vi "周期任务设置.vi"(11 "TimingControl 输入":refnum<class "TimingControl.lvclass">) -> (3 "TimingControl 输出":refnum<class "TimingControl.lvclass">)   [LabVIEW 2016, in "TimingControl.lvlib" / "TimingControl.lvclass"]
uses:
  TimingControl.lvclass
  <vilib>/Utility/miscctls.llb/LVPointTypeDef.ctl
  TimingControl.lvclass/TimingControl.ctl
panel:
  in  "保存":bool
  in  "退出":bool
  in  "添加":bool
  in  "删除":bool
  in  "清空":bool
  in  "任务列表":i32(listbox)
  out "启动次数":i32
  out "测试状态.启动时间":timestamp caption="启动时间" format="%<%y/%m/%d %H:%M:%S>T"
  in  "每日启动":T1
  in  "每周启动":T2
  in  "每月启动":T3
  in  "控制命令":T4
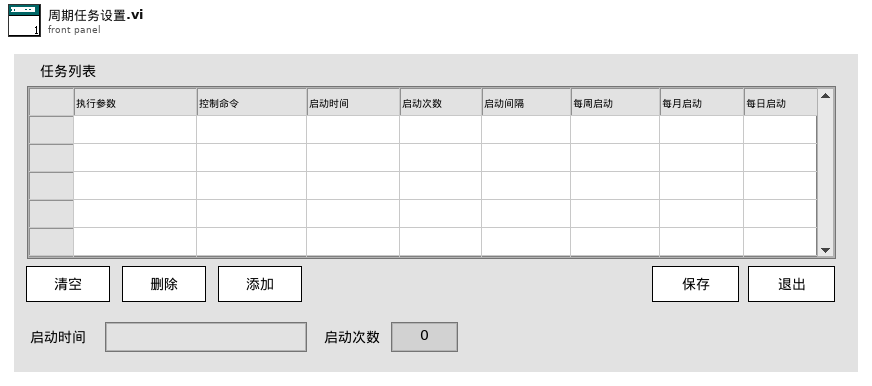
[diagram p1: front panel]
types:
  T1 = typedef "TimingControl.lvlib/TimingControl.lvclass/每日启动.ctl" = enum16{"关闭", "每日"}
  T2 = typedef "TimingControl.lvlib/TimingControl.lvclass/每周启动.ctl" = enum16{"关闭", "周日", "周一", "周二", "周三", "周四", "周五", "周六"}
  T3 = typedef "TimingControl.lvlib/TimingControl.lvclass/每月启动.ctl" = enum16{"关闭", "1号", "2号", "3号", "4号", "5号", "6号", "7号", "8号", "9号", "10号", "11号", "12号", "13号", "14号", "15号", "16号", "17号", "18号", "19号", "20号", "21号", "22号", "23号", "24号", "25号", "26号", "27号", "28号", "29号", "30号", "31号"}
  T4 = typedef "TimingControl.lvlib/TimingControl.lvclass/国标控制命令.ctl" = enum16{"启动测量", "标样核查", "零点核查", "跨度核查", "空白测试", "平行样测试", "加标回收", "空白校准", "标样校准", "初始化（清洗）", "停止测试", "仪器重启", "校时", "模式设置", "测量间隔设置"}
  T5 = typedef "LVPointTypeDef.ctl" = cluster{"Horizontal":i16, "Vertical":i16}
  T6 = typedef "TimingControl.lvlib/TimingControl.lvclass/State Data.ctl" = cluster{"仪器时间":timestamp, "仪器运行状态":bool, "配置文件路径":path, "测量参数":T7, "测试状态":cluster{"启动时间":timestamp, "结束时间":timestamp, "启动次数":i32}, "配置信息":T8}
  T7 = typedef "TimingControl.lvlib/TimingControl.lvclass/测量参数.ctl" = cluster{"测量参数":string[]}
  T8 = typedef "TimingControl.lvlib/TimingControl.lvclass/配置信息.ctl" = cluster{"每周启动":T2, "每月启动":T3, "周期模式":T9, "测量参数":T7, "定点周期":T10, "间隔启动":T12, "配置时间":timestamp, "配置":cluster{"测量参数":string, "控制命令":T4, "启动时间":string, "启动次数":u16, "启动间隔":dbl, "每周启动":T2, "每月启动":T3, "每日启动":enum16{"关闭", "每日"}}[]}
  T9 = typedef "TimingControl.lvlib/TimingControl.lvclass/周期模式设置.ctl" = enum16{"定点模式", "间隔模式"}
  T10 = typedef "TimingControl.lvlib/TimingControl.lvclass/定点周期设置.ctl" = cluster{"时间":u16, "启动命令":T11}
  T11 = typedef "TimingControl.lvlib/TimingControl.lvclass/启动命令选择.ctl" = enum16{"", "水样测试", "标样核查", "零点核查", "跨度核查", "空白测试", "平行样测试", "加标回收", "空白校准", "标样校准", "初始化(清洗)"}
  T12 = typedef "TimingControl.lvlib/TimingControl.lvclass/间隔启动设置.ctl" = cluster{"启动命令":T11, "启动间隔":dbl, "启动次数":i32}
  T13 = cluster{"测量参数":string, "控制命令":T4, "启动时间":string, "启动次数":u16, "启动间隔":dbl, "每周启动":T2, "每月启动":T3, "每日启动":enum16{"关闭", "每日"}}[]
  T14 = cluster{string, "index of element":i32, string, i32, dbl, "index of element":i32, "index of element":i32, "index of element":i32}
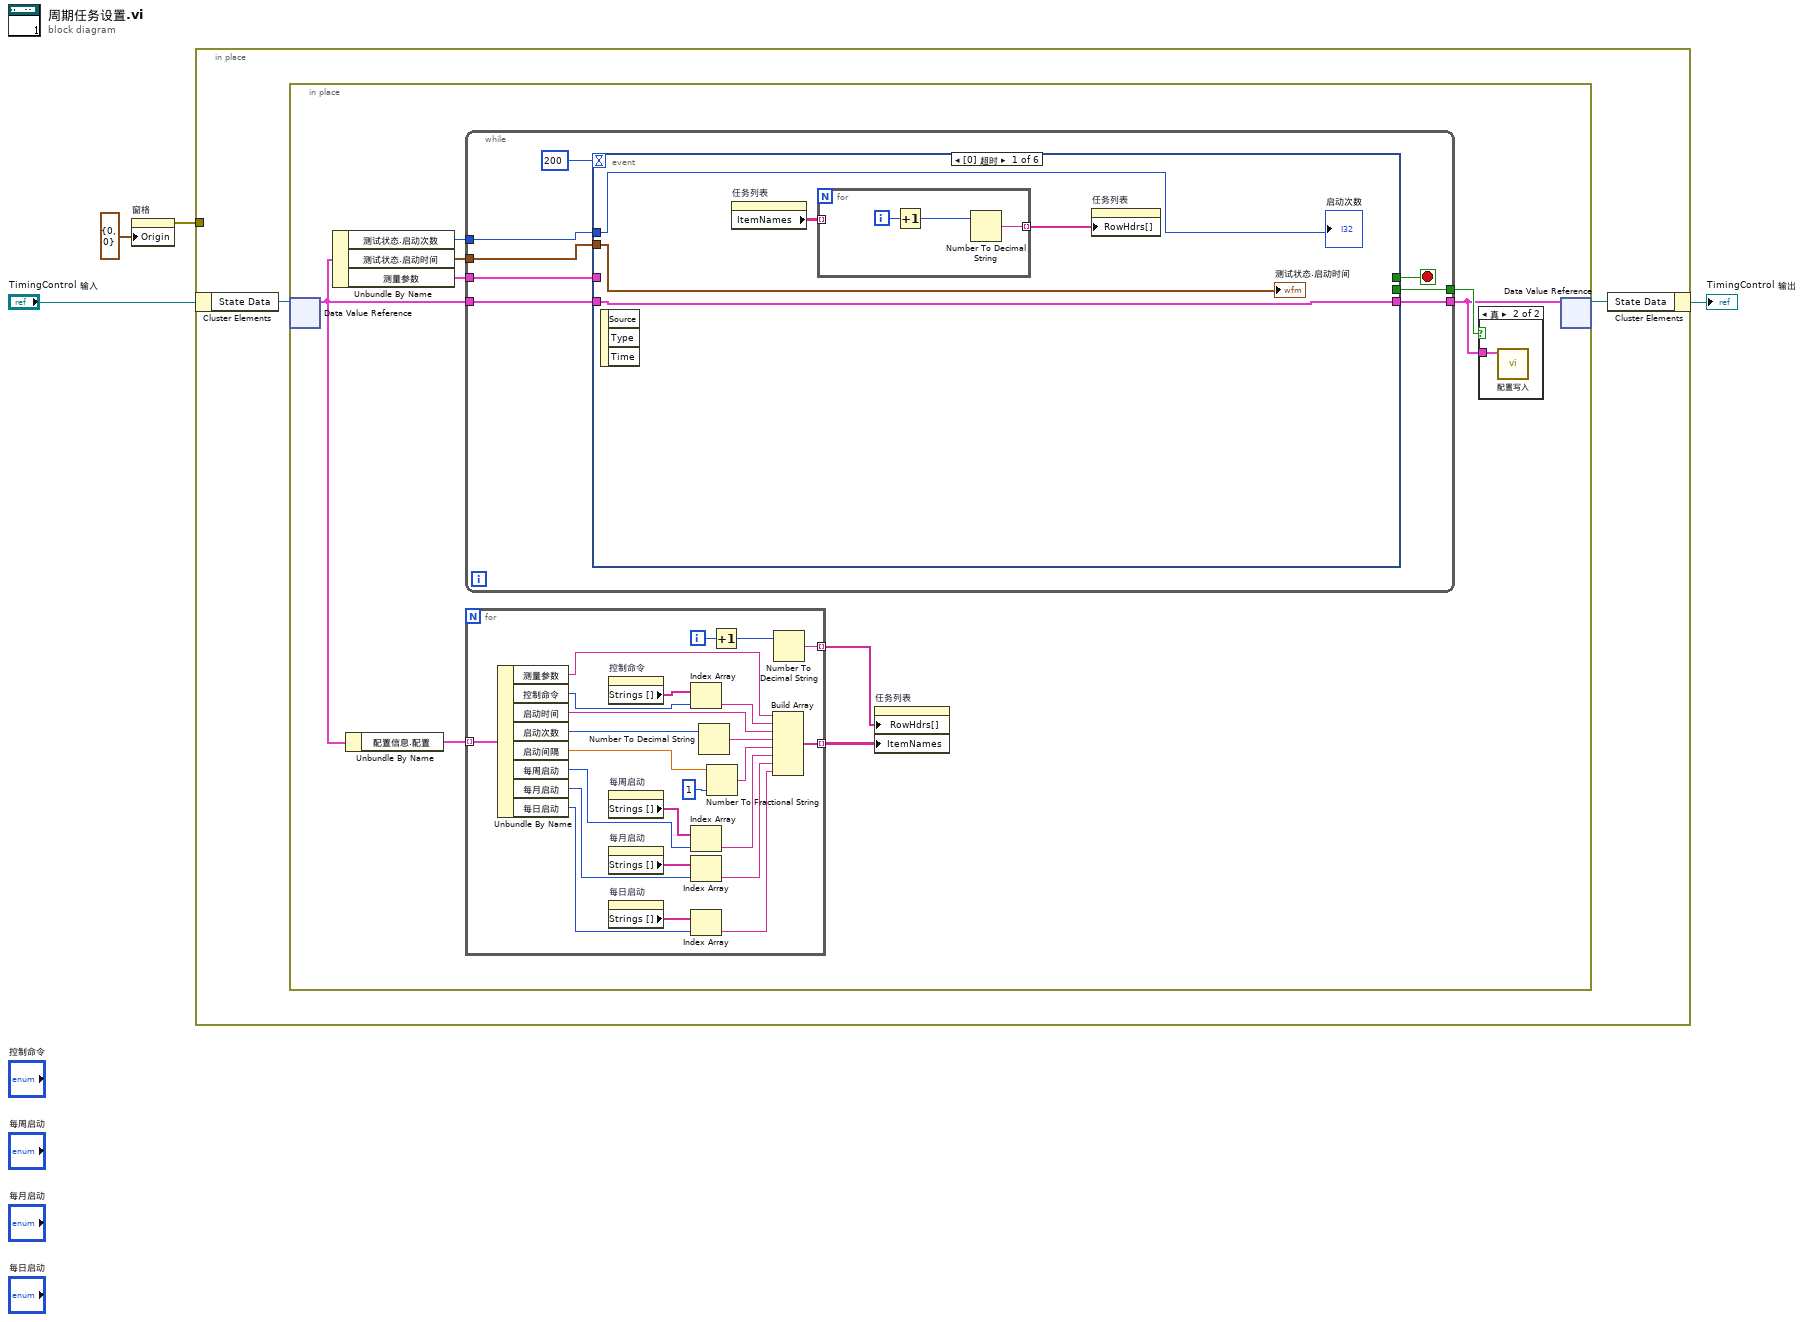
[diagram p0: block diagram]
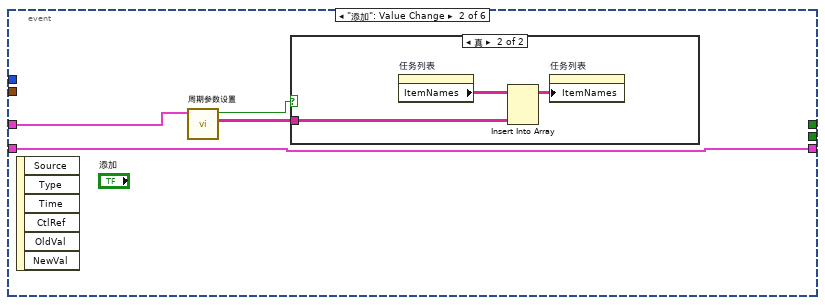
[diagram p3: hidden frame]
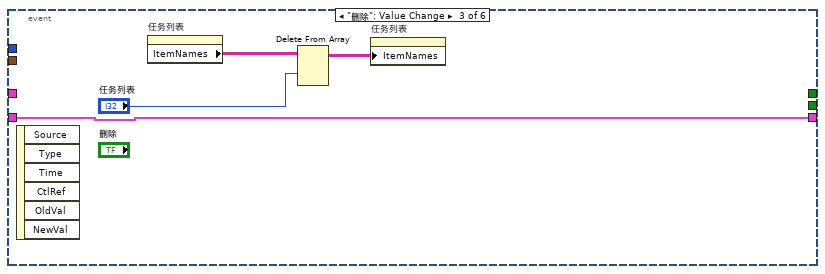
[diagram p5: hidden frame]
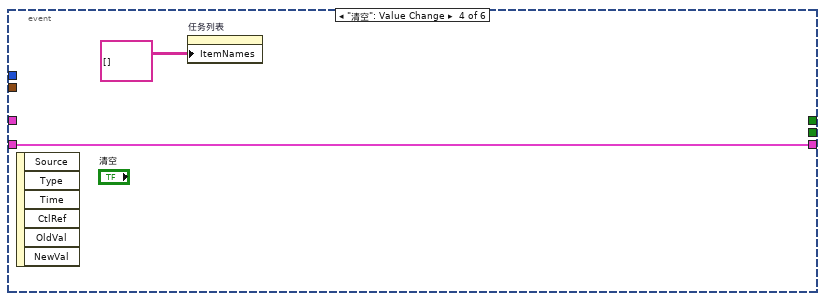
[diagram p6: hidden frame]
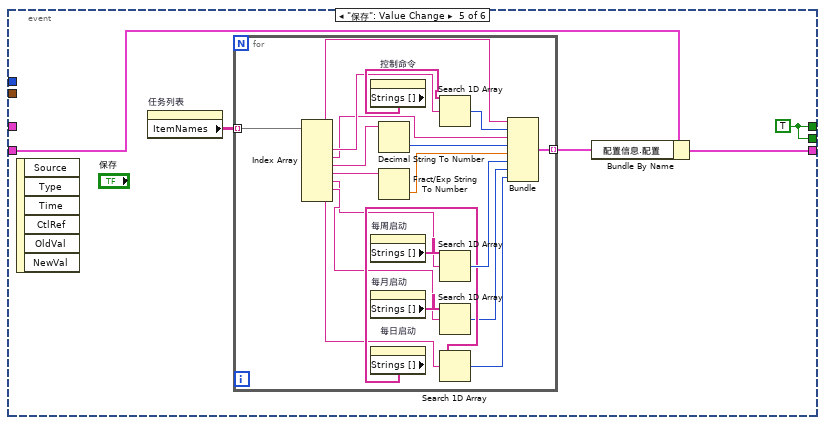
[diagram p7: hidden frame]
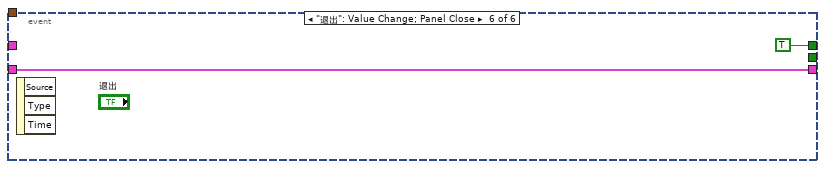
[diagram p8: hidden frame]
diagram:
  n1 = property on="窗格" class="Pane"("Origin"=T5 {"Horizontal"=0, "Vertical"=0} ("原点")) -> (error out=w1:errorcluster)  [unwired: 2 in, 1 out]
  n2 = in-place {
    in-place-border: w1 -> [_]
    n3 = in-place-cluster #1("TimingControl 输入") -> ("State Data"=w6:refnum<data-value>)
    n4 = in-place {
      n5 = in-place-dvr #2(w6) -> (w7:T6)  [unwired: 1 out]
      n6 = Unbundle By Name(w7) -> ("测试状态.启动次数"=w11:i32, "测试状态.启动时间"=w12:timestamp, "测量参数"=w15:T7)
      n7 = Unbundle By Name(w7) -> ("配置信息.配置"=w8:T13)
      n8 = while {
        tunnel: w15 -> [w48]
        tunnel: w7 -> [w46]
        tunnel: [w45] -> w13
        tunnel: [w43] -> w14
        tunnel: w12 -> [w42]
        tunnel: w11 -> [w41]
        stop <- w44 stop-if-true
        n9 = event shown="[0] 超时" {
          selector: _ -> [_ _ _ _ _ _]
          dyn-events: _ -> [_ _ _ _ _ _]
          timeout: 200 -> [_ _ _ _ _ _]
          tunnel: [_ _ _ _ w74 TRUE] -> w44
          tunnel: w48 -> [_ w58 _ _ _ _]
          tunnel: w46 -> [w53 w57 w67 w69 w72 w95]
          tunnel: [w53 w57 w67 w69 w70 w95] -> w45
          tunnel: [_ _ _ _ w74 _] -> w43
          tunnel: w42 -> [w50 _ _ _ _ _]
          tunnel: w41 -> [w49 _ _ _ _ _]
          event Timeout {
            n10 = event-data() -> ()  [unwired: 1 in, 3 out]
            n11 = property on="任务列表" class="MCListbox (严格)"() -> ("ItemNames"=w51:string[][])  [unwired: 2 in, 2 out]
            n12 = for {
              tunnel: w51 -> [_] mode=indexing
              tunnel: [w54] -> w52 mode=indexing
              i -> [w55]
              n13 = Increment(x=w55) -> (x+1=w56:i32)
              n14 = Number To Decimal String(number=w56) -> (decimal integer string=w54:string)  [unwired: 1 in]
            }
            n15 = property on="任务列表" class="MCListbox (严格)"("RowHdrs[]"=w52) -> ()  [unwired: 2 in, 2 out]
            "测试状态.启动时间" <- w50
            "启动次数" <- w49
          }
          event "添加": Value Change {
            n16 = event-data() -> ()  [unwired: 1 in, 6 out]
            n17 = call "周期参数设置.vi"("测量参数输入"=w58) -> ("数组"=w59:string[][], "输出"=w60:bool)  [unwired: 9 in]
            n18 = case shown="真" w60 {
              tunnel: w59 -> [_ w62]
              frame False {
              }
              frame True {
                n19 = property on="任务列表" class="MCListbox (严格)"() -> ("ItemNames"=w63:string[][])  [unwired: 2 in, 2 out]
                n20 = Insert Into Array(array=w63, new element=w62) -> (w61:string[][])  [unwired: 2 in]
                n21 = property on="任务列表" class="MCListbox (严格)"("ItemNames"=w61) -> ()  [unwired: 2 in, 2 out]
              }
            }
          }
          event "删除": Value Change {
            n22 = event-data() -> ()  [unwired: 1 in, 6 out]
            n23 = property on="任务列表" class="MCListbox (严格)"() -> ("ItemNames"=w66:string[][])  [unwired: 2 in, 2 out]
            n24 = Delete From Array(array=w66, index (row)="任务列表") -> (array with subset deleted=w64:string[][])  [unwired: 2 in, 1 out]
            n25 = property on="任务列表" class="MCListbox (严格)"("ItemNames"=w64) -> ()  [unwired: 2 in, 2 out]
          }
          event "清空": Value Change {
            n26 = event-data() -> ()  [unwired: 1 in, 6 out]
            n27 = property on="任务列表" class="MCListbox (严格)"("ItemNames"=string[][] [] ("项名")) -> ()  [unwired: 2 in, 2 out]
          }
          event "保存": Value Change {
            w74 = TRUE
            n28 = event-data() -> ()  [unwired: 1 in, 6 out]
            n29 = property on="任务列表" class="MCListbox (严格)"() -> ("ItemNames"=w73:string[][])  [unwired: 2 in, 2 out]
            n30 = for {
              tunnel: w73 -> [w94] mode=indexing
              tunnel: [w82] -> w71 mode=indexing
              n31 = Index Array(array=w94) -> (element #1=w93:string, element #2=w91:string, element #3=w89:string, element #4=w76:string, element #5=w78:string, element #6=w79:string, element #7=w80:string, element #8=w81:string)  [unwired: 8 in]
              n32 = property on="控制命令" class="Enum (严格)"() -> ("Strings []"=w92:string[])  [unwired: 2 in, 2 out]
              n33 = property on="每周启动" class="Enum (严格)"() -> ("Strings []"=w88:string[])  [unwired: 2 in, 2 out]
              n34 = property on="每月启动" class="Enum (严格)"() -> ("Strings []"=w86:string[])  [unwired: 2 in, 2 out]
              n35 = property on="每日启动" class="Enum (严格)"() -> ("Strings []"=w85:string[])  [unwired: 2 in, 2 out]
              n36 = Decimal String To Number(string=w76) -> (number=w75:i32)  [unwired: 2 in, 1 out]
              n37 = Fract/Exp String To Number(string=w78) -> (number=w77:dbl)  [unwired: 3 in, 1 out]
              n38 = Search 1D Array(1D array=w92, element=w91) -> (index of element=w90:i32)  [unwired: 1 in]
              n39 = Search 1D Array(1D array=w88, element=w79) -> (index of element=w87:i32)  [unwired: 1 in]
              n40 = Search 1D Array(1D array=w86, element=w80) -> (index of element=w84:i32)  [unwired: 1 in]
              n41 = Search 1D Array(1D array=w85, element=w81) -> (index of element=w83:i32)  [unwired: 1 in]
              n42 = Bundle(w93, "index of element"=w90, w89, w75, w77, "index of element"=w87, "index of element"=w84, "index of element"=w83) -> (w82:T14)  [unwired: 1 in]
            }
            n43 = Bundle By Name(cluster=w72, "配置信息.配置"=w71) -> (w70:T6)
          }
          event "退出": Value Change; Panel Close {
            n44 = event-data() -> ()  [unwired: 1 in, 3 out]
          }
        }
      }
      n45 = for {
        tunnel: w8 -> [w39] mode=indexing
        tunnel: [w36] -> w9 mode=indexing
        tunnel: [w16] -> w10 mode=indexing
        i -> [w37]
        n46 = Unbundle By Name(w39) -> ("测量参数"=w35:string, "控制命令"=w33:T4, "启动时间"=w31:string, "启动次数"=w30:u16, "启动间隔"=w28:dbl, "每周启动"=w25:T2, "每月启动"=w21:T3, "每日启动"=w19:enum16{"关闭", "每日"})
        n47 = property on="控制命令" class="Enum (严格)"() -> ("Strings []"=w34:string[])  [unwired: 2 in, 2 out]
        n48 = property on="每周启动" class="Enum (严格)"() -> ("Strings []"=w24:string[])  [unwired: 2 in, 2 out]
        n49 = property on="每月启动" class="Enum (严格)"() -> ("Strings []"=w22:string[])  [unwired: 2 in, 2 out]
        n50 = property on="每日启动" class="Enum (严格)"() -> ("Strings []"=w20:string[])  [unwired: 2 in, 2 out]
        n51 = Index Array(array=w34, index=w33) -> (element=w32:string)
        n52 = Index Array(array=w24, index=w25) -> (element=w23:string)
        n53 = Index Array(array=w22, index=w21) -> (element=w18:string)
        n54 = Index Array(array=w20, index=w19) -> (element=w17:string)
        n55 = Number To Decimal String(number=w30) -> (decimal integer string=w29:string)  [unwired: 1 in]
        n56 = Number To Fractional String(number=w28, precision (6)=i16 1 ("精度(6)")) -> (F-format string=w27:string)  [unwired: 2 in]
        n57 = Increment(x=w37) -> (x+1=w38:i32)
        n58 = Build Array(w35, w32, w31, w29, w27, w23, w18, w17) -> (w16:string[])
        n59 = Number To Decimal String(number=w38) -> (decimal integer string=w36:string)  [unwired: 1 in]
      }
      n60 = property on="任务列表" class="MCListbox (严格)"("RowHdrs[]"=w9, "ItemNames"=w10) -> ()  [unwired: 2 in, 2 out]
      n61 = case shown="真" w14 {
        tunnel: w13 -> [_ w40]
        frame False {
        }
        frame True {
          n62 = call "配置写入.vi"("数据值"=w40) -> ()  [unwired: 10 in, 1 out]
        }
      }
      n63 = in-place-dvr #2(w13) -> (w5:refnum<data-value>)  [unwired: 1 out]
    }
    n64 = in-place-cluster #1("State Data"=w5) -> (→"TimingControl 输出":refnum<class "TimingControl.lvclass">)
  }
